vi "LAS-CTS_NDFilterScan.vi"() -> ()   [LabVIEW 2024]
uses:
  <vilib>/httpClient/LabVIEWHTTPClient.lvlib
  <vilib>/Analysis/NI_AALBase.lvlib
panel:
  out "Ion Current Chart":dbl(graph)
  out "Average Ion Current (pA)":dbl format="%.3g"
  in  "Ammeter Range":dbl(ring)=0.02 items=["20 mA"=0.02, "2 mA"=0.002, "200 uA"=0.0002, "20 uA"=2e-05, "2 uA"=2e-06, "200 nA"=2e-07, "20 nA"=2e-08, "2 nA"=2e-09, "200 pA"=2e-10, "20 pA"=2e-11]
  in  "Keithly":refnum<visa-resource-name>
  out "Laser Energy Chart":dbl(graph)
  out "Average Laser Energy (uJ)":dbl format="%.3g"
  out "ND Filter Position":i32
  in  "file path (use dialog)":path
  in  "# of Positions":i32
  in  "Step Size":i32
  in  "ND Filter":refnum<visa-resource-name>
  in  "Number of Pulses":i32
  out "number of measurements":i32
  out "Laser Energy (uJ)":dbl
  in  "Energy Meter":refnum<visa-resource-name>
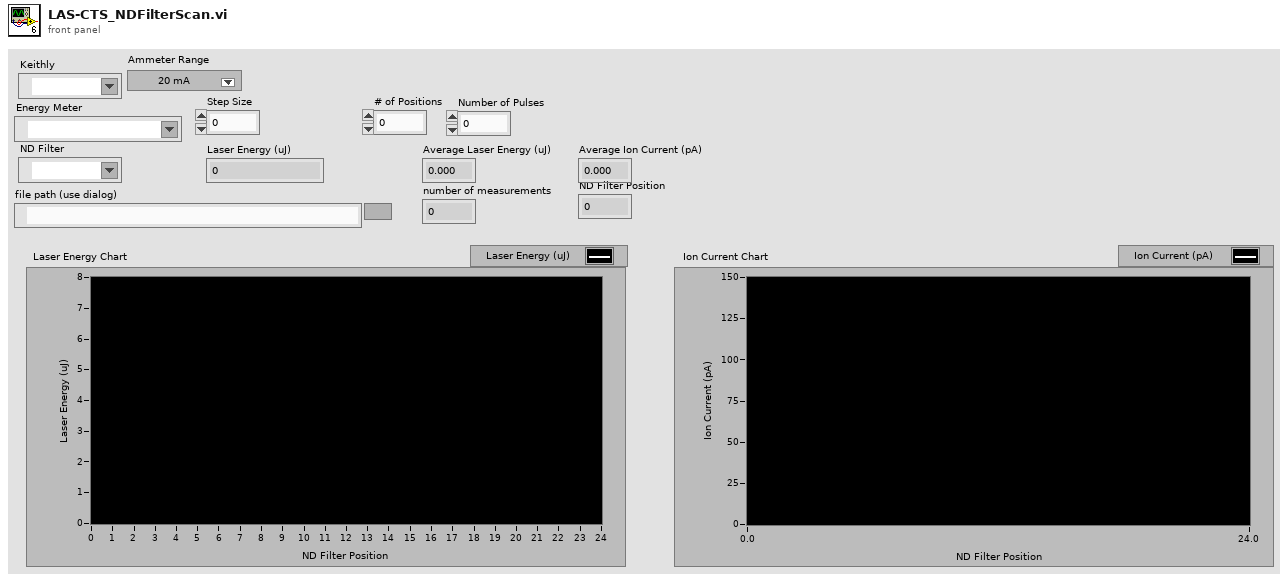
[diagram p1: front panel]
types:
  T1 = enum16{"open", "replace", "create", "open or create", "replace or create", "replace or create with confirmation"}
  T2 = typedef "LabVIEWHTTPClient.lvlib/ClientHandle.ctl" = refnum<k1>
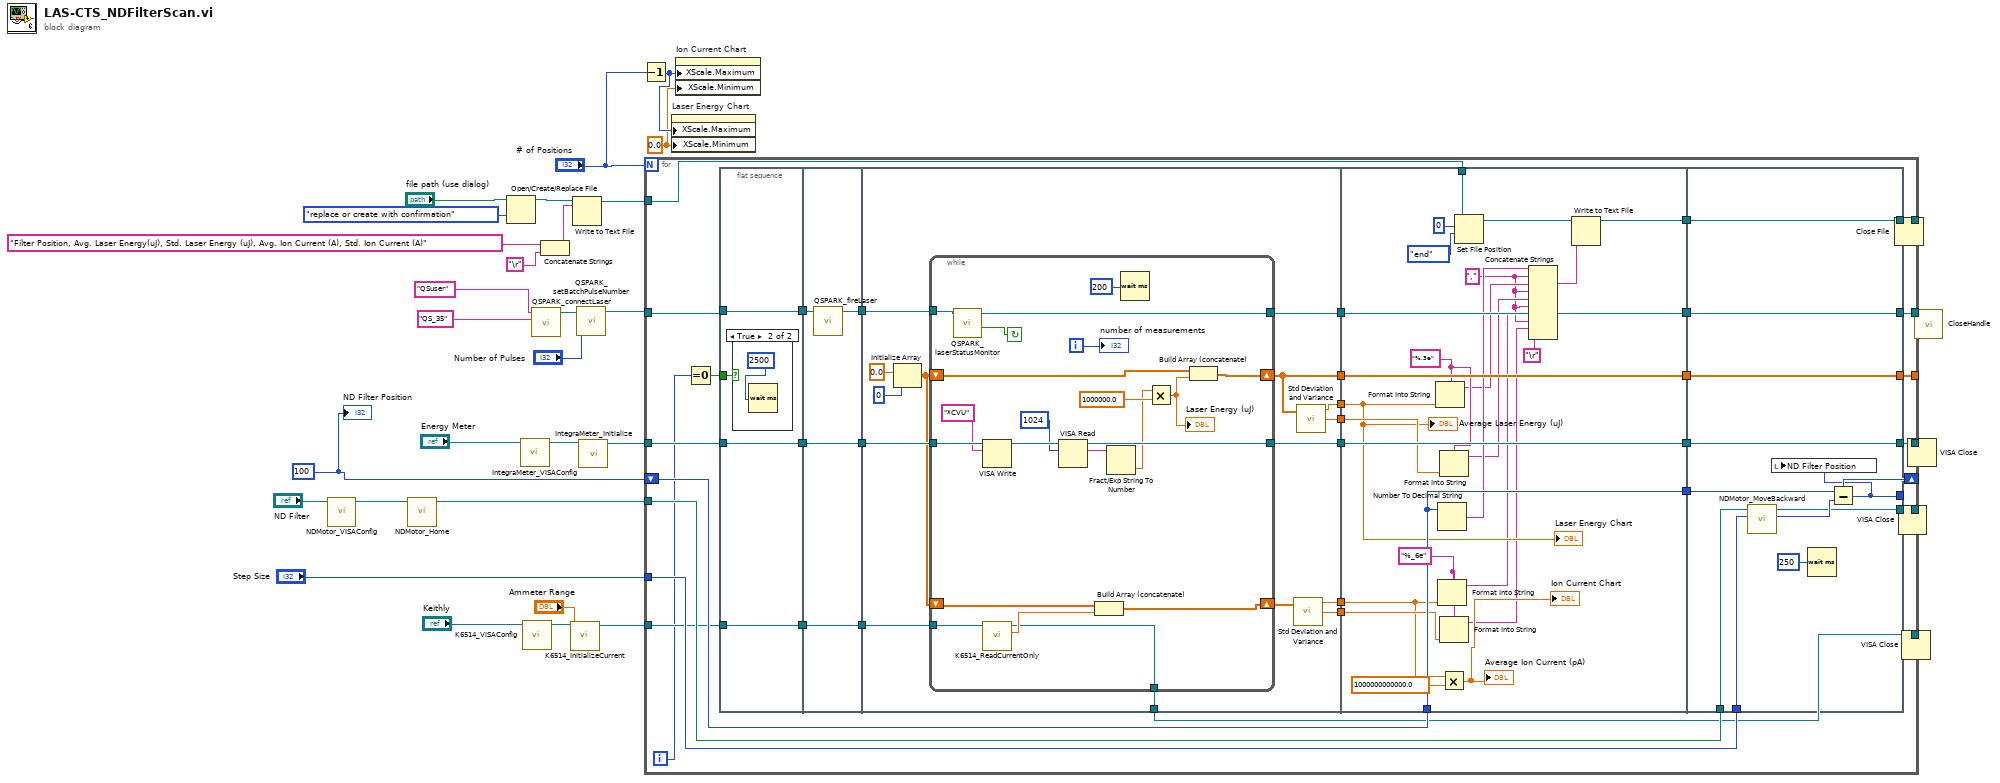
[diagram p0: block diagram]
diagram:
  w1 = 100 ("Start Position")
  w2 = 0.0 ("X Scale.Range:Minimum")
  n1 = call "NDMotor_VISAConfig.vi"("VISA resource name"="ND Filter") -> ("reference out"=w21:refnum<visa-resource-name>)  [unwired: 9 in, 1 out]
  n2 = call "NDMotor_Home.vi"("VISA resource name"=w21) -> ("VISA resource name out"=w20:refnum<visa-resource-name>)  [unwired: 9 in, 1 out]
  n3 = Open/Create/Replace File(file path (use dialog)="file path (use dialog)", operation (0:open)=T1."replace or create with confirmation") -> (refnum out=w13:refnum<file>)  [unwired: 4 in, 2 out]
  n4 = call "IntegraMeter_VISAConfig.vi"("VISA resource name"="Energy Meter") -> ("reference out"=w32:refnum<visa-resource-name>)  [unwired: 9 in, 1 out]
  n5 = call "K6514_VISAConfig.vi"("VISA resource name"="Keithly") -> ("reference out"=w8:refnum<visa-resource-name>)  [unwired: 9 in, 1 out]
  n6 = call "QSPARK_connectLaser.vi"("password"="QS_35", "username"="QSuser") -> ("client handle out"=w25:T2)  [unwired: 9 in]
  n7 = Concatenate Strings("Filter Position, Avg. Laser Energy(uJ), Std. Laser Energy (uJ), Avg. Ion Current (A), Std. Ion Current (A)" ("text"), "\r") -> (w16:string)
  n8 = call "K6514_InitializeCurrent.vi"("Range"="Ammeter Range", "VISA resource name"=w8) -> ("VISA resource name out"=w6:refnum<visa-resource-name>)  [unwired: 8 in, 1 out]
  n9 = Write to Text File(file (use dialog)=w13, text=w16) -> (refnum out=w15:refnum<file>)  [unwired: 2 in, 2 out]
  n10 = call "QSPARK_setBatchPulseNumber.vi"("Number of Pulses"="Number of Pulses", "client handle"=w25) -> ("client handle out"=w28:T2)  [unwired: 9 in]
  n11 = call "IntegraMeter_Initialize.vi"("VISA resource name"=w32) -> ("VISA resource name out"=w30:refnum<visa-resource-name>)  [unwired: 9 in, 1 out]
  n12 = Decrement(x="# of Positions") -> (x-1=w3:i32)
  n13 = for {
    N: "# of Positions" -> [_]
    tunnel: [w60] -> _
    tunnel: "Step Size" -> [w47]
    tunnel: w15 -> [w56]
    tunnel: w28 -> [w62]
    tunnel: [w61] -> w26
    tunnel: w30 -> [w64]
    tunnel: [w63] -> w29
    tunnel: w20 -> [w45]
    tunnel: [w55] -> w14
    shift-right: [w54] -> _
    shift-left: w1 -> [w53]
    tunnel: [w46] -> w10
    tunnel: w6 -> [w41]
    tunnel: [w38] -> w5
    i -> [w33]
    n14 = Equal To 0?(x=w33) -> (x = 0?=w34:bool)
    n15 = flat-sequence {
      tunnel: w41 -> [w68]
      tunnel: w64 -> [w69]
      tunnel: w62 -> [w70]
      tunnel: [w70] -> w37
      tunnel: [w69] -> w36
      tunnel: [w68] -> w35
      tunnel: w34 -> [w67]
      tunnel: [w75] -> w66
      tunnel: [w73] -> w65
      tunnel: [w72] -> w42
      tunnel: w37 -> [w74]
      tunnel: w36 -> [w75]
      tunnel: w35 -> [w72]
      tunnel: w66 -> [w90]
      tunnel: w65 -> [w88]
      tunnel: [w89] -> w59
      tunnel: [w87] -> w58
      tunnel: [w84] -> w57
      tunnel: [w83] -> w44
      tunnel: [w82] -> w43
      tunnel: w42 -> [w81]
      tunnel: [w78] -> w40
      tunnel: [w77] -> w39
      tunnel: [w76] -> w38
      tunnel: w59 -> [w136]
      tunnel: w58 -> [w135]
      tunnel: w57 -> [w134]
      tunnel: w56 -> [w131]
      tunnel: w53 -> [w127]
      tunnel: [w136] -> w52
      tunnel: [w135] -> w51
      tunnel: [w134] -> w50
      tunnel: [w129] -> w49
      tunnel: [w127] -> w48
      tunnel: w44 -> [w117]
      tunnel: w43 -> [w125]
      tunnel: w40 -> [w118]
      tunnel: w39 -> [w121]
      tunnel: [w138] -> w54
      tunnel: [w144] -> w55
      tunnel: [w145] -> w60
      tunnel: [w146] -> w61
      tunnel: [w147] -> w63
      tunnel: w52 -> [w147]
      tunnel: w51 -> [w146]
      tunnel: w50 -> [w145]
      tunnel: w49 -> [w144]
      tunnel: w48 -> [w142]
      tunnel: w47 -> [w141]
      tunnel: [w140] -> w46
      tunnel: w45 -> [w139]
      frame #0 {
        n16 = case shown="True" w67 {
          frame False {
          }
          frame True {
            n17 = Wait (ms)(milliseconds to wait=2500) -> ()  [unwired: 1 out]
          }
        }
      }
      frame #1 {
        n18 = call "QSPARK_fireLaser.vi"("client handle"=w74) -> ("client handle out"=w73:T2)  [unwired: 10 in]
      }
      frame #2 {
        n19 = Initialize Array(0.0 ("element"), 0 ("dimension size")) -> (w80:dbl[])
        n20 = while {
          tunnel: w90 -> [w111]
          tunnel: [w109] -> w89
          tunnel: w88 -> [w104]
          tunnel: [w103] -> w87
          shift-right: [w100] -> w84
          shift-left: w80 -> [w101]
          tunnel: w81 -> [w92]
          shift-right: [w94] -> w79
          shift-left: w80 -> [w95]
          tunnel: [w91] -> w76
          i -> [w105]
          stop <- w102 continue-if-true
          n21 = call "QSPARK_laserStatusMonitor.vi"("client handle"=w104) -> ("laser on?"=w102:bool, "client handle out"=w103:T2)  [unwired: 8 in, 1 out]
          n22 = VISA Write(VISA resource name=w111, write buffer="*CVU") -> (VISA resource name out=w110:refnum<visa-resource-name>)  [unwired: 1 in, 2 out]
          n23 = call "K6514_ReadCurrentOnly.vi"("VISA resource name"=w92) -> ("Current (A)"=w93:dbl, "VISA resource name out"=w91:refnum<visa-resource-name>)  [unwired: 6 in, 2 out]
          n24 = VISA Read(VISA resource name=w110, byte count=u32 1024) -> (VISA resource name out=w109:refnum<visa-resource-name>, read buffer=w106:string)  [unwired: 1 in, 2 out]
          n25 = Build Array (concatenate)(w95, w93) -> (w94:dbl[])
          n26 = Fract/Exp String To Number(string=w106) -> (number=w97:dbl)  [unwired: 3 in, 1 out]
          n27 = Wait (ms)(milliseconds to wait=u32 200 ("millisecond multiple")) -> ()  [unwired: 1 out]
          n28 = Multiply(x=w97, y=1000000.0) -> (x*y=w96:dbl)
          "Laser Energy (uJ)" <- w96
          n29 = Build Array (concatenate)(w101, w96) -> (w100:dbl[])
          "number of measurements" <- w105
        }
        n30 = call <vilib>:"Std Deviation and Variance.vi"("X"=w79) -> ("mean"=w78:dbl, "standard deviation"=w77:dbl)  [unwired: 1 in, 1 out]
        n31 = call <vilib>:"Std Deviation and Variance.vi"("X"=w84) -> ("mean"=w83:dbl, "standard deviation"=w82:dbl)  [unwired: 1 in, 1 out]
      }
      frame #3 {
        w120 = "%_6e" ("format string")
        w113 = "," ("string")
        w126 = "%.3e" ("format string")
        n32 = Format Into String(format string=w126, w117) -> (resulting string=w123:string)  [unwired: 2 in, 1 out]
        n33 = Number To Decimal String(number=w127) -> (decimal integer string=w124:string)  [unwired: 1 in]
        n34 = Format Into String(format string=w120, w118) -> (resulting string=w115:string)  [unwired: 2 in, 1 out]
        n35 = Format Into String(format string=w126, w125) -> (resulting string=w122:string)  [unwired: 2 in, 1 out]
        n36 = Format Into String(format string=w120, w121) -> (resulting string=w114:string)  [unwired: 2 in, 1 out]
        n37 = Multiply(x=w118, y=1000000000000.0) -> (x*y=→"Average Ion Current (pA)" →"Ion Current Chart":dbl)
        n38 = Set File Position(offset (in bytes) (0)=i64 0, refnum=w131, from (0:start)=enum16{"start", "end", "current"}."end") -> (refnum out=w130:refnum<file>)  [unwired: 1 in, 1 out]
        n39 = Concatenate Strings(w124, w113, w123, w113, w122, w113, w115, w113, w114, "\r") -> (w128:string)
        n40 = Write to Text File(file (use dialog)=w130, text=w128) -> (refnum out=w129:refnum<file>)  [unwired: 2 in, 2 out]
        "Average Laser Energy (uJ)" <- w117
        "Laser Energy Chart" <- w117
      }
      frame #4 {
        n41 = call "NDMotor_MoveBackward.vi"("Steps"=w141, "VISA resource name"=w139) -> ("steps"=w143:i32, "VISA resource name out"=w140:refnum<visa-resource-name>)  [unwired: 6 in, 2 out]
        n42 = Wait (ms)(milliseconds to wait=u32 250) -> ()  [unwired: 1 out]
        n43 = Subtract(x=w142, y=w143) -> (x-y=w138:i32)
        n44 = local write "ND Filter Position"(w138) -> ()
      }
    }
  }
  n45 = property on="Laser Energy Chart" class="WFChart (strict)"("XScale.Maximum"=w3, "XScale.Minimum"=w2) -> ()  [unwired: 2 in, 2 out]
  n46 = property on="Ion Current Chart" class="WFChart (strict)"("XScale.Maximum"=w3, "XScale.Minimum"=w2) -> ()  [unwired: 2 in, 2 out]
  n47 = Close File(refnum=w14) -> ()  [unwired: 1 in, 2 out]
  n48 = VISA Close(VISA resource name=w10) -> ()  [unwired: 1 in, 1 out]
  n49 = VISA Close(VISA resource name=w5) -> ()  [unwired: 1 in, 1 out]
  n50 = VISA Close(VISA resource name=w29) -> ()  [unwired: 1 in, 1 out]
  n51 = call <vilib>:"CloseHandle.vi"("client handle"=w26) -> ()  [unwired: 14 in, 1 out]
  "ND Filter Position" <- w1
